vi "reSizeSplitter-FW.vi"(0 "this vi":refnum<vi>, 1 "pane":refnum<vi>, 2 "left":i16=-1, 3 "top":i16=-1, 5 "Width":u32, 7 "Height":u32, 12 "pane2":refnum<vi>) -> (4 "reference out":refnum<vi>)   [LabVIEW 2013]
uses:
  <vilib>/Utility/miscctls.llb/LVRectTypeDef.ctl
panel:
  out "Front Panel Window:Panel Bounds":T1
  in  "Height 2":u32
  out "output cluster":T1
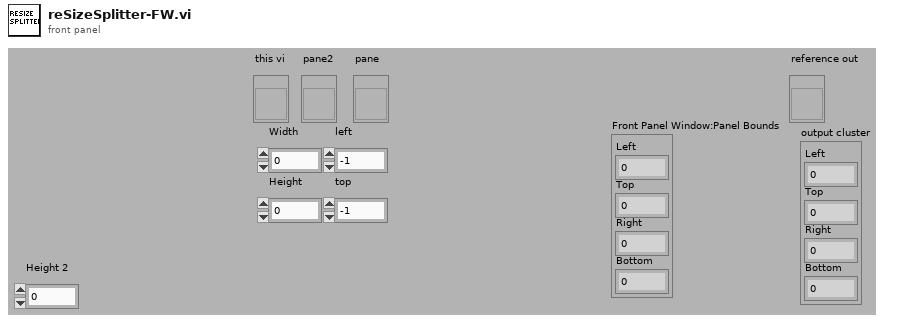
[diagram p1: front panel]
types:
  T1 = typedef "LVRectTypeDef.ctl" = cluster{"Left":i16, "Top":i16, "Right":i16, "Bottom":i16}
  T2 = typedef "LVBoundsTypeDef.ctl" = cluster{"Width":u32, "Height":u32}
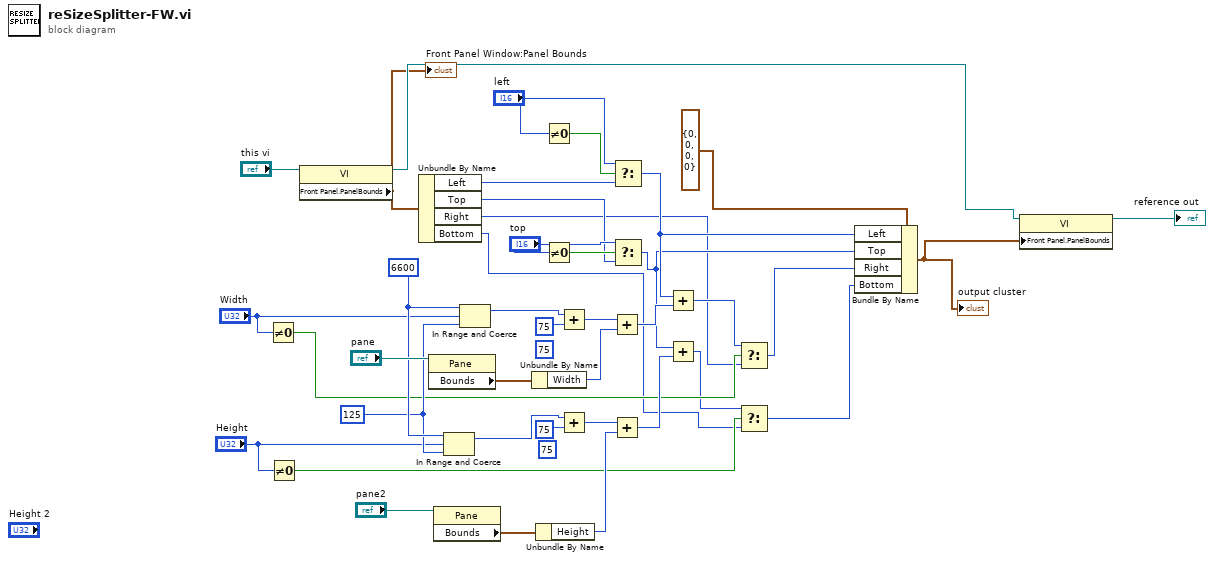
[diagram p0: block diagram]
diagram:
  (unwired) u32 75 ("y")
  (unwired) u32 75 ("y")
  w18 = u32 125 ("lower limit")
  w19 = u32 6600 ("upper limit")
  n1 = Not Equal To 0?(x="Width") -> (x != 0?=w8:bool)
  n2 = Not Equal To 0?(x="Height") -> (x != 0?=w4:bool)
  n3 = property class="VI"(reference="this vi") -> (reference out=w27:refnum<vi>, "Front Panel.PanelBounds"=w26:T1)  [unwired: 1 in, 1 out]
  "Front Panel Window:Panel Bounds" <- w26
  n4 = Unbundle By Name(w26) -> ("Left"=w12:i16, "Top"=w11:i16, "Right"=w6:i16, "Bottom"=w2:i16)
  n5 = property class="Pane"(reference="pane") -> ("Bounds"=w40:T2)  [unwired: 1 in, 2 out]
  n6 = property class="Pane"(reference="pane2") -> ("Bounds"=w39:T2)  [unwired: 1 in, 2 out]
  n7 = In Range and Coerce(upper limit=w19, x="Height", lower limit=w18) -> (coerced(x)=w17:u32)  [unwired: 1 out]
  n8 = In Range and Coerce(upper limit=w19, x="Width", lower limit=w18) -> (coerced(x)=w20:u32)  [unwired: 1 out]
  n9 = Unbundle By Name(w40) -> ("Width"=w33:u32)
  n10 = Unbundle By Name(w39) -> ("Height"=w38:u32)
  n11 = Not Equal To 0?(x="left") -> (x != 0?=w22:bool)
  n12 = Not Equal To 0?(x="top") -> (x != 0?=w21:bool)
  n13 = Add(x=w20, y=u32 75) -> (x+y=w30:u32)
  n14 = Add(x=w17, y=u32 75) -> (x+y=w29:u32)
  n15 = Add(x=w30, y=w33) -> (x+y=w36:u32)
  n16 = Add(x=w29, y=w38) -> (x+y=w35:u32)
  n17 = Select(t="left", s=w22, f=w12) -> (s? t:f=w14:i16)
  n18 = Select(t="top", s=w21, f=w11) -> (s? t:f=w13:i16)
  n19 = Add(x=w14, y=w36) -> (x+y=w7:u32)
  n20 = Add(x=w13, y=w35) -> (x+y=w3:u32)
  n21 = Select(t=w7, s=w8, f=w6) -> (s? t:f=w5:u32)
  n22 = Select(t=w3, s=w4, f=w2) -> (s? t:f=w1:u32)
  n23 = Bundle By Name(cluster=T1 {"Left"=0, "Top"=0, "Right"=0, "Bottom"=0} ("Front Panel Window:Panel Bounds"), "Left"=w14, "Top"=w13, "Right"=w5, "Bottom"=w1) -> (w34:T1)
  "output cluster" <- w34
  n24 = property class="VI"(reference=w27, "Front Panel.PanelBounds"=w34) -> (reference out=→"reference out":refnum<vi>)  [unwired: 1 in, 1 out]
